vi "Read Geode Robots.vi"(11 "Mine in":refnum<class "Mine.lvclass">) -> (2 "Geode Robots":u8, 3 "Mine out":refnum<class "Mine.lvclass">)   [LabVIEW 2023, in "d19.lvlib" / "Mine.lvclass"]
uses:
  Mine.lvclass
  Mine.lvclass/Mine.ctl
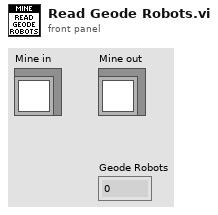
[diagram p1: front panel]
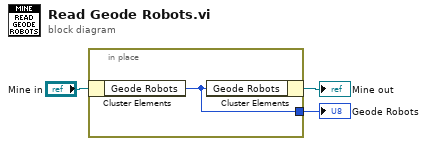
[diagram p0: block diagram]
diagram:
  n1 = in-place {
    in-place-border: [w4] -> w3
    n2 = in-place-cluster #1("Mine in") -> ("Geode Robots"=w4:u8)
    n3 = in-place-cluster #1("Geode Robots"=w4) -> (→"Mine out":refnum<class "Mine.lvclass">)
  }
  "Geode Robots" <- w3
